vi "Arcade Strafe.vi"(8 "error in":errorcluster, 9 "dt (s)":dbl, 10 "Deadzone":dbl=0.15 format="%#_13g", 11 "Left Joystick X":dbl) -> (0 "error out":errorcluster, 3 "Strafe Output":dbl)   [LabVIEW 2014]
doc: "Controls strafing. Has deadzone and ramping implemented via BypassControl.\nInputs:\n Prev Value - The previous strafe motor value\n Left Joystick X - The value of the strafe motor controlling joystick\n Strafe Ramp - Determines how quickly the strafe should be allowed to accelerate, set at DashBoard\nOutputs:\n Strafe Output - The modified motor output to be sent to the strafe motor"
uses:
  <vilib>/Rock Robotics/WPI/MotorControl/WPI_MotorControlDeviceRef.ctl
  <vilib>/Rock Robotics/WPI/MotorControl/WPI_MotorControlType.ctl
  <vilib>/Rock Robotics/SystemInterfaces/Typedef/FPGA_TypedefDigitalModule.ctl
  <vilib>/Rock Robotics/SystemInterfaces/DIO/FPGA_DIOPWMChannel.ctl
  <vilib>/Rock Robotics/WPI/PWM/WPI_PWMDeadband.ctl
  <vilib>/Rock Robotics/WPI/CAN/Jaguar/SubVIs/WPI_CANJaguar_ControlMode.ctl
  <vilib>/Rock Robotics/WPI/CAN/TalonSRX/WPI_CANTalonSRX_APIControlMode.ctl
  <vilib>/Rock Robotics/WPI/PWM/WPI_PWMTransform_ConPane.ctl
  <vilib>/Rock Robotics/Network Tables/SD Read Number.vi
panel:
  in  "Strafe Ref":T1={"DeviceStatus"={"status"=FALSE, "code"=0, "source"=""}, "Type"=enum."PWM", "PWM"={"Controller"=enum."Controller 1", "PWM Channel"=enum."Invalid", "DeadBand"={"Name"="", "maxPositivePwm"=0, "minPositivePwm"=0, "centerPwm"=0, "maxNegativePwm"=0, "minNegativePwm"=0, "angularRange"=0}}, "CAN"={"Device Number"=0, "Control Mode"=enum."Percent VBus", "Semaphore"=refnum, "Max Vout"=12.0, "TalonSRX Control Mode"=enum."Percent VBus"}, "Invert"=FALSE, "TransformRef"=refnum, "InvTransformRef"=refnum}
  in  "Time":dbl
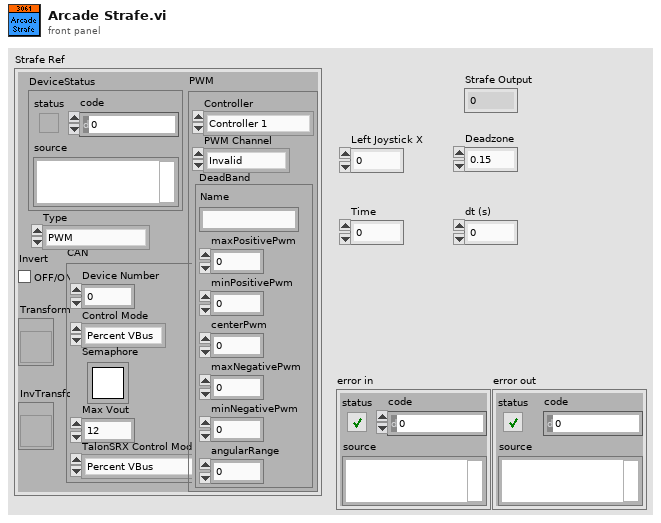
[diagram p1: front panel]
types:
  T1 = typedef "WPI_MotorControlDeviceRef.ctl" = cluster{"DeviceStatus":errorcluster, "Type":T2, "PWM":cluster{"Controller":T3, "PWM Channel":T4, "DeadBand":T5}, "CAN":cluster{"Device Number":u8, "Control Mode":T6, "Semaphore":T7, "Max Vout":dbl, "TalonSRX Control Mode":T8}, "Invert":bool, "TransformRef":T9, "InvTransformRef":T9}
  T2 = typedef "WPI_MotorControlType.ctl" = enum16{"PWM", "CAN", "CANTalonSRX"}
  T3 = typedef "FPGA_TypedefDigitalModule.ctl" = enum16{"Controller 1"}
  T4 = typedef "FPGA_DIOPWMChannel.ctl" = enum8{"PWM 0", "PWM 1", "PWM 2", "PWM 3", "PWM 4", "PWM 5", "PWM 6", "PWM 7", "PWM 8", "PWM 9", "PWM MXP 0", "PWM MXP 1", "PWM MXP 2", "PWM MXP 3", "PWM MXP 4", "PWM MXP 5", "PWM MXP 6", "PWM MXP 7", "PWM MXP 8", "PWM MXP 9", "Invalid"}
  T5 = typedef "WPI_PWMDeadband.ctl" = cluster{"Name":string, "maxPositivePwm":i32, "minPositivePwm":i32, "centerPwm":i32, "maxNegativePwm":i32, "minNegativePwm":i32, "angularRange":u16}
  T6 = typedef "WPI_CANJaguar_ControlMode.ctl" = enum8{"Percent VBus", "Current", "Speed", "Position", "Voltage"}
  T7 = typedef "Semaphore RefNum" = refnum<k1>
  T8 = typedef "WPI_CANTalonSRX_APIControlMode.ctl" = enum8{"Percent VBus", "Speed", "Position", "Slave", "Unchanged / Invalid"}
  T9 = typedef "WPI_PWMTransform_ConPane.ctl" = refnum<vi>
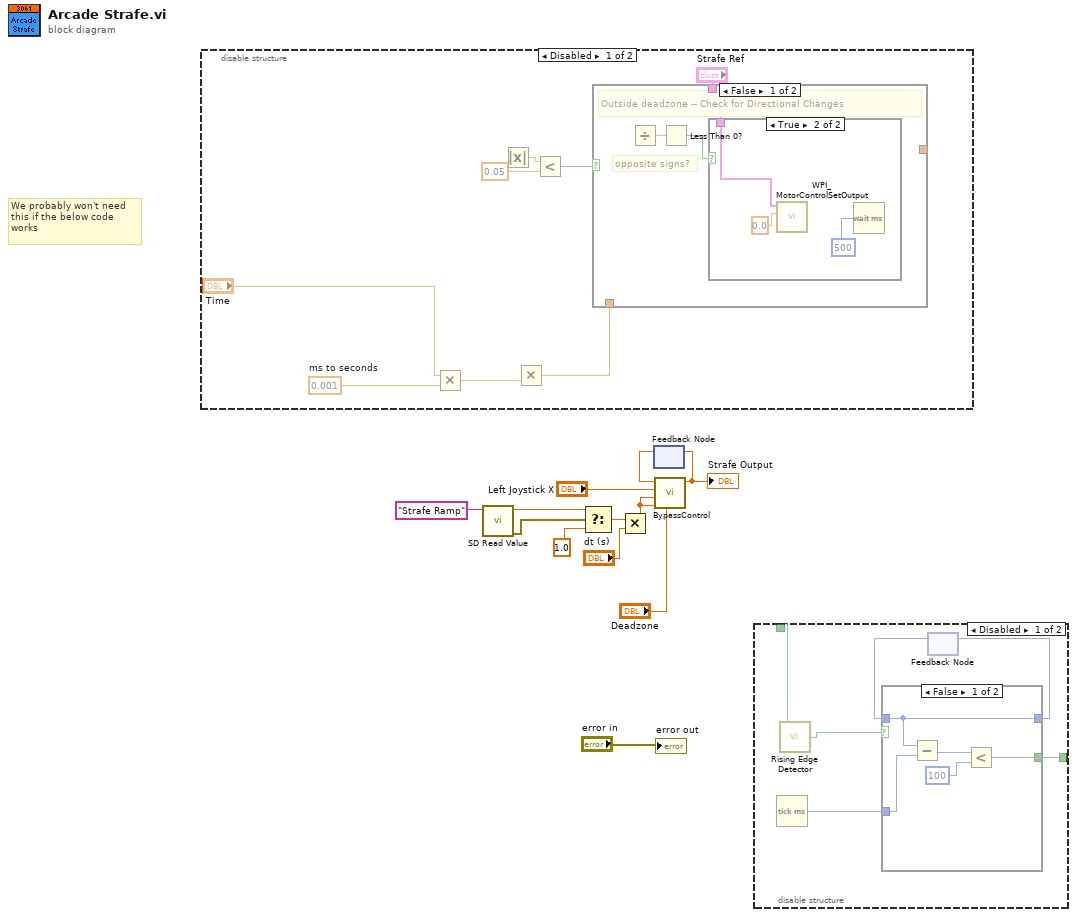
[diagram p0: block diagram]
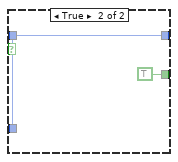
[diagram p2: hidden frame]
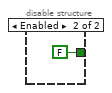
[diagram p3: hidden frame]
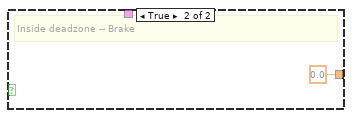
[diagram p5: hidden frame]
diagram:
  # "We probably won't need\nthis if the below code\nworks"
  n1 = disable-structure shown="Disabled" {
    frame Disabled {
      w21 = 0.001  # ms to seconds
      n2 = Multiply(x="Time", y=w21) -> (x*y=w20:dbl)
      n3 = Absolute Value() -> (abs(x)=w16:dbl)  [unwired: 1 in]
      n4 = Multiply(y=w20) -> (x=w18:dbl, x*y=w17:dbl)
      n5 = Less?(x=w16, y=0.05) -> (x < y?=w14:bool)
      n6 = case shown="False" w14 {
        tunnel: w17 -> [_ _]
        tunnel: [_ 0.0 ("Left Joystick X")] -> _
        tunnel: "Strafe Ref" -> [w22 _]
        frame False {
          # "opposite signs?"
          # "Outside deadzone -- Check for Directional Changes"
          n7 = Divide() -> (x/y=w24:dbl)  [unwired: 2 in]
          n8 = Less Than 0?(x=w24) -> (x < 0?=w23:bool)
          n9 = case shown="True" w23 {
            tunnel: w22 -> [_ w27]
            frame False {
            }
            frame True {
              n10 = call <vilib>:"WPI_MotorControlSetOutput.vi"("Output"=0.0, "MotorControlDevRef"=w27) -> ()  [unwired: 7 in, 3 out]
              n11 = Wait (ms)(milliseconds to wait=u32 500) -> ()  [unwired: 1 out]
            }
          }
        }
        frame True {
          # "Inside deadzone -- Brake"
        }
      }
    }
    frame Enabled {
    }
  }
  n12 = call-poly <vilib>:"SD Read Value.vi"("Name"="Strafe Ramp") -> ("error out"=w9:errorcluster, "Numeric"=w8:dbl)  [unwired: 8 in, 1 out]
  n13 = Select(t=w8, s=w9, f=1.0 ("t")) -> (s? t:f=w3:dbl)
  n14 = Multiply(x=w3, y="dt (s)") -> (x*y=w1:dbl)
  n15 = feedback #1() -> (w5:dbl)  [unwired: 1 in]
  n16 = call "BypassControl.vi"("Cutoff"="Deadzone", "MaxMotorChangeForward"=w1, "MaxMotorChangeBackward"=w1, "Current Input"="Left Joystick X", "Previous Input"=w5) -> ("SetMotor"=w4:dbl)  [unwired: 5 in, 1 out]
  "Strafe Output" <- w4
  n17 = feedback-in #1(w4) -> ()
  n18 = disable-structure shown="Disabled" {
    disable-tunnel: _ -> [w34 _]
    disable-tunnel: [w29 FALSE] -> _
    frame Disabled {
      n19 = Tick Count (ms)() -> (millisecond timer value=w32:u32)
      n20 = call "Rising Edge Detector.vi"("Input"=w34) -> ("Rising edge?"=w33:bool)
      n21 = feedback #2() -> (w30:u32)  [unwired: 1 in]
      n22 = case shown="False" w33 {
        tunnel: [w38 w41] -> w31
        tunnel: w32 -> [w39 w41]
        tunnel: w30 -> [w38 _]
        tunnel: [w36 TRUE] -> w29
        frame False {
          n23 = Subtract(x=w38, y=w39) -> (x-y=w37:u32)
          n24 = Less?(x=w37, y=u32 100) -> (x < y?=w36:bool)
        }
        frame True {
        }
      }
      n25 = feedback-in #2(w31) -> ()
    }
    frame Enabled {
    }
  }
  "error out" <- "error in"
